vi "Limits Page.vi"(8 "error in (no error)":errorcluster, 10 "LBCB Number":T2) -> (0 "error out":errorcluster)   [LabVIEW 2009]
uses:
  lib/Limits/Limit Slider.ctl
  lib/Data Access Objects/Metadata/LBCB Number.ctl
  lib/Data Access Objects/Limits/DofTypes.ctl
  lib/Limits/Slider Messages.ctl
  lib/Control Loop/Parameters Changes.ctl
  lib/Control Loop/Parameter Change States.ctl
  lib/Data Access Objects/Metadata/Persistant DAO Actions.ctl
  lib/Data Access Objects/Application/Number Of LBCBs.ctl
  lib/Limits/Faults List Actions.ctl
  lib/Limits/Lower Upper Select.ctl
  lib/Launcher/NoPanelAppTypes.ctl
  lib/Launcher/Launcher Actions.ctl
panel:
  out "Messages":string
  in  "Ok":bool
  in  "DofType":T1
  in  "Limit Slider 6":T3 {"Slide" scale=-0.3..0.3 scale format="%#_6f"}
  in  "Limit Slider 5":T3 {"Slide" scale=-0.3..0.3 scale format="%#_6f"}
  in  "Limit Slider 4":T3 {"Slide" scale=-0.3..0.3 scale format="%#_6f"}
  in  "Limit Slider 3":T3 {"Slide" scale=-1.0..1.0 scale format="%#_6f"}
  in  "Limit Slider 2":T3 {"Slide" scale=-1.0..1.0 scale format="%#_6f"}
  in  "Limit Slider 1":T3 {"Slide" scale=-1.0..1.0 scale format="%#_6f"}
  # "Lower"
  # "Higher"
  # "Current"
  # "Global"
  # "Local"
  # "Lower"
  # "Higher"
  # "Current"
  # "Global"
  # "Local"
  # "Lower"
  # "Higher"
  # "Current"
  # "Global"
  # "Local"
  # "Lower"
  # "Higher"
  # "Current"
  # "Global"
  # "Local"
  # "Lower"
  # "Higher"
  # "Current"
  # "Global"
  # "Local"
  # "Lower"
  # "Higher"
  # "Current"
  # "Global"
  # "Local"
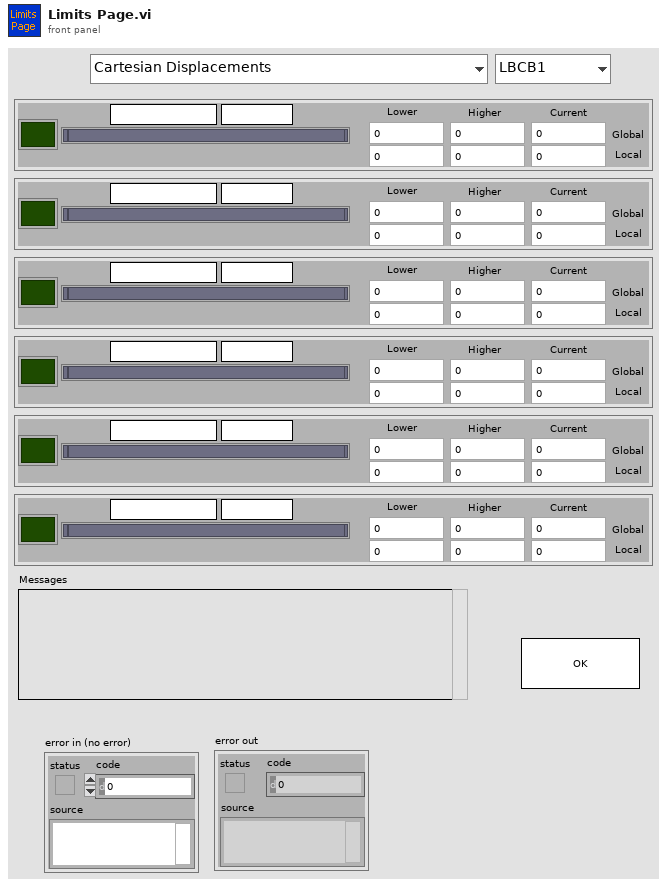
[diagram p1: front panel]
types:
  T1 = typedef "DofTypes.ctl" = enum16{"Cartesian Displacements", "Cartesian Forces & Moments", "Actuator Displacements", "Actuator Forces"}
  T2 = typedef "LBCB Number.ctl" = enum16{"LBCB1", "LBCB2"}
  T3 = typedef "Limit Slider.ctl" = cluster{"Slide":cluster{dbl, dbl, dbl, dbl}, "Global Lo":dbl, "Global Hi":dbl, "Local Lo":dbl, "Local Hi":dbl, "Fault":bool, "DofLabel":string, "Units":string, "Global Actual":dbl, "Local Actual":dbl}
  T4 = typedef "Parameters Changes.ctl" = cluster{"Change State":T5, "LBCB Number":T2}
  T5 = typedef "Parameter Change States.ctl" = enum16{"Mixed Mode", "Control Loop", "Limits", "Application", "Stiffness Jacobian", "Start DAQ", "Reset Auto-Balance", "Set Command", "Enable Control", "Disable Control", "Position", "Stop Application"}
  T6 = typedef "Slider Messages.ctl" = enum16{"Update Display", "Exit", "Nothing"}
  T7 = typedef "Persistant DAO Actions.ctl" = enum16{"Init", "Get", "Set", "Load", "Save"}
  T8 = enum8{"Enabled", "Disabled", "Disabled and Grayed Out"}
  T9 = typedef "Number Of LBCBs.ctl" = enum16{"1", "2"}
  T10 = typedef "Faults List Actions.ctl" = enum16{"Init", "Add", "Remove", "Get List"}
  T11 = typedef "Lower Upper Select.ctl" = enum16{"Lower", "Upper"}
  T12 = typedef "Fault Id.ctl" = cluster{"Fault Type":T13, "LBCB Number":T2, "Index":u32, "Space Type":T14}
  T13 = typedef "Fault Type.ctl" = enum16{"None", "Command", "Displacement", "Force", "Increment"}
  T14 = typedef "Space Type.ctl" = enum16{"Actuator", "Cartesian"}
  T15 = cluster{"[0]":dbl, "[1]":dbl, "[2]":dbl, "[3]":dbl, "[4]":dbl, "[5]":dbl, "[6]":dbl, "[7]":dbl, "[8]":dbl}[]
  T16 = cluster{"[0]":dbl, "[1]":dbl, "[2]":dbl, "[3]":dbl, "[4]":dbl, "[5]":dbl, "[6]":dbl, "[7]":dbl, "[8]":dbl}
  T17 = cluster{"[0]":dbl, "[1]":dbl, "[2]":dbl, "[3]":dbl}
  T18 = typedef "NoPanelAppTypes.ctl" = enum16{"NTCP Socket", "Data Archiving", "DAQ Link", "Control Loops", "Cmd Disp Diffs", "Connection Offsets", "Limits", "Increment Limits"}
  T19 = typedef "Launcher Actions.ctl" = enum16{"Launch", "Stop All", "Stop", "Kill", "Running?", "Init"}
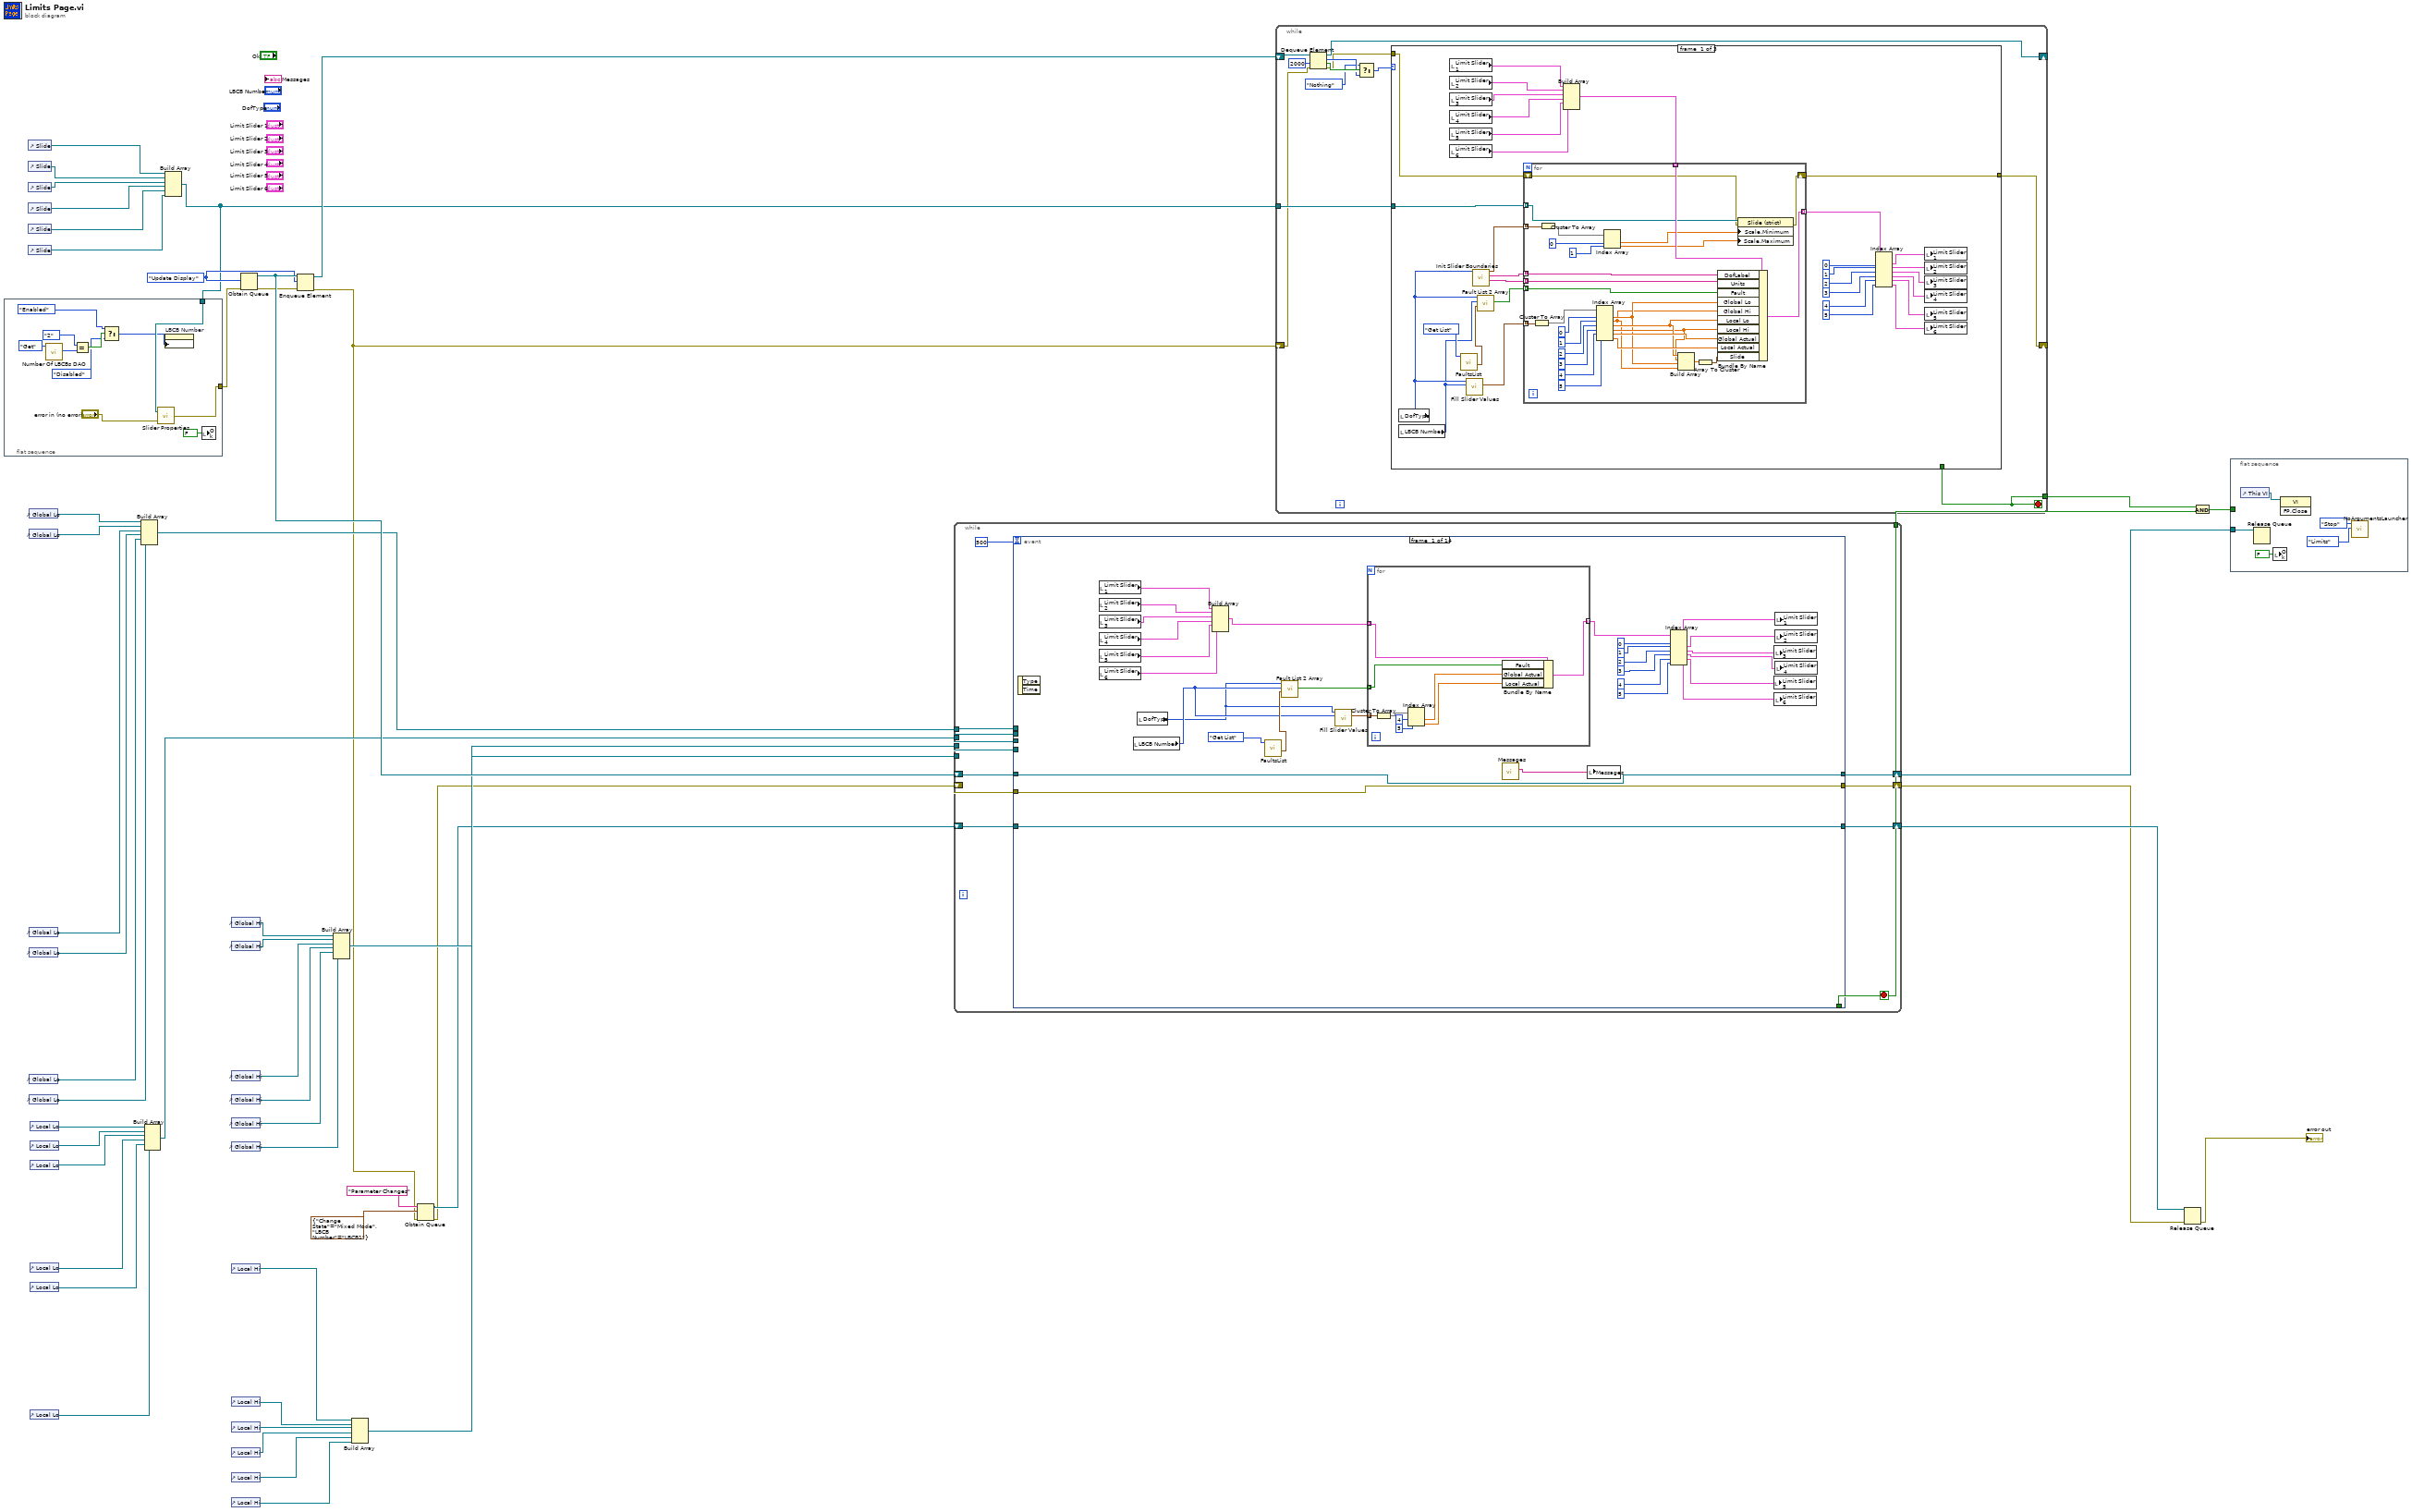
[diagram p0: block diagram]
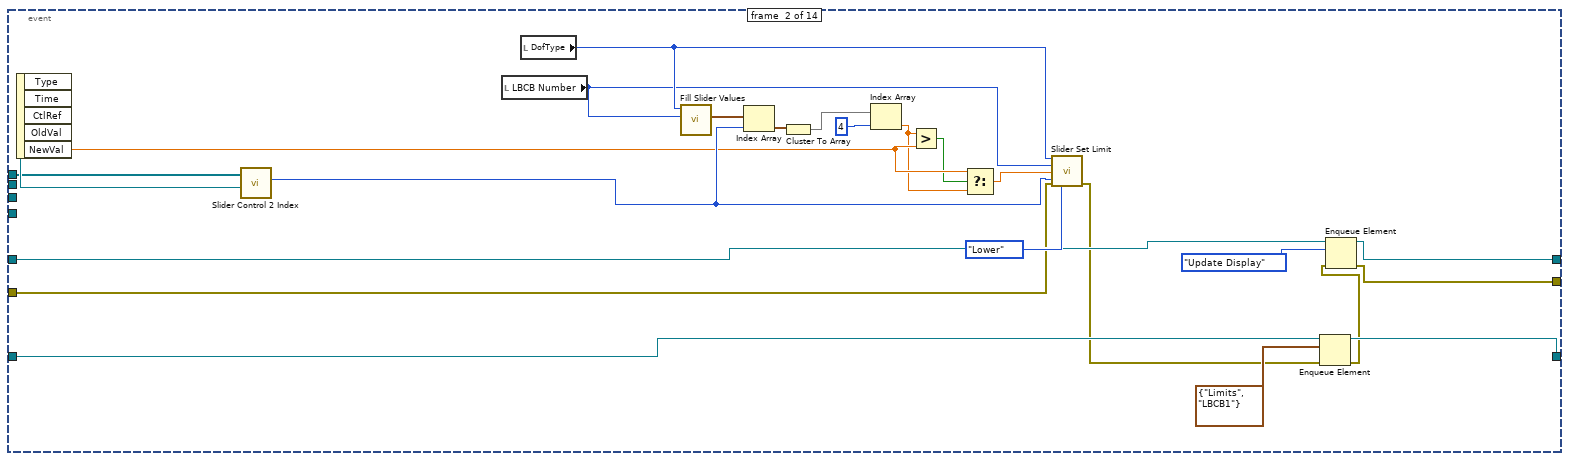
[diagram p2: hidden frame]
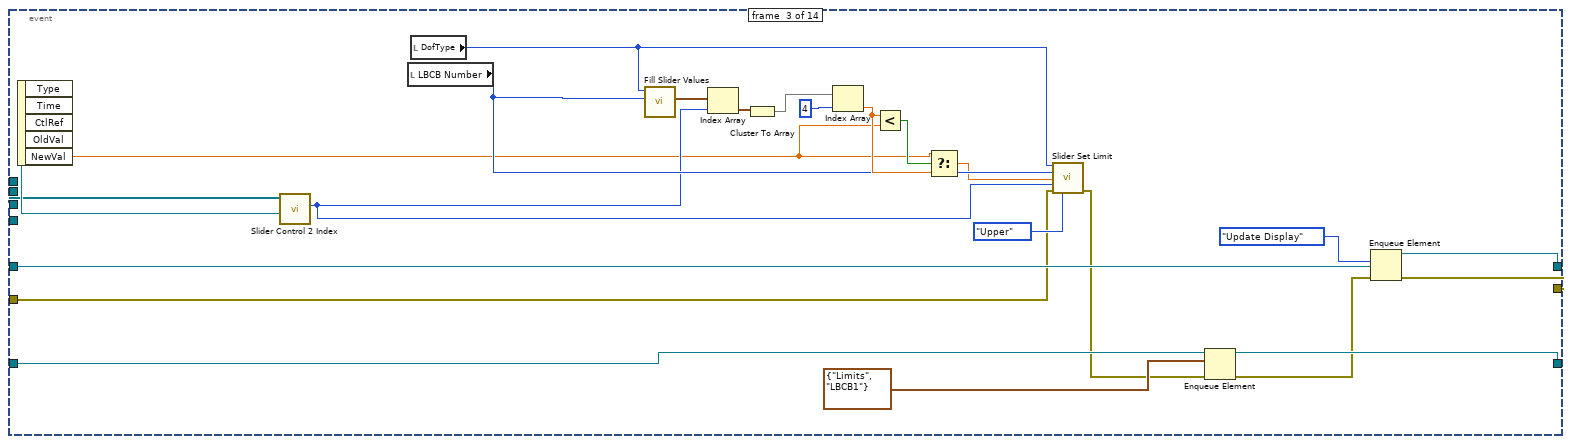
[diagram p3: hidden frame]
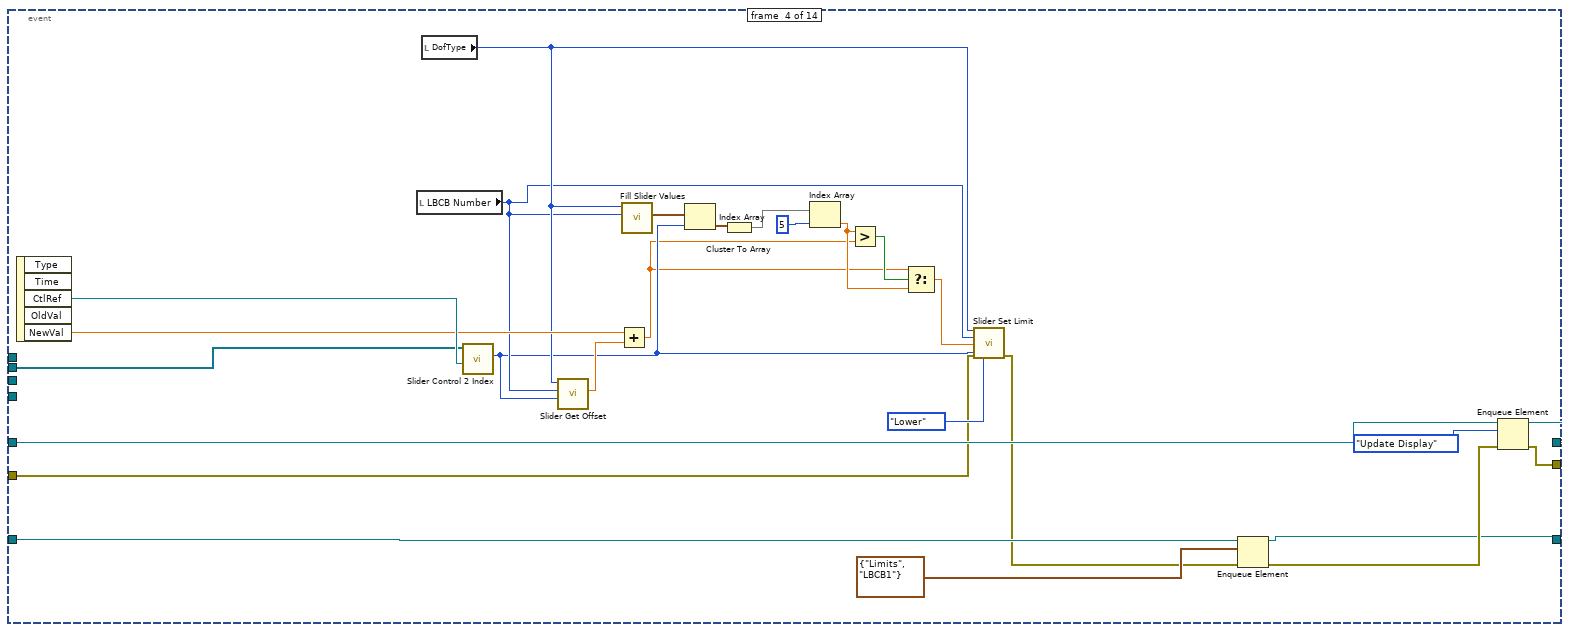
[diagram p4: hidden frame]
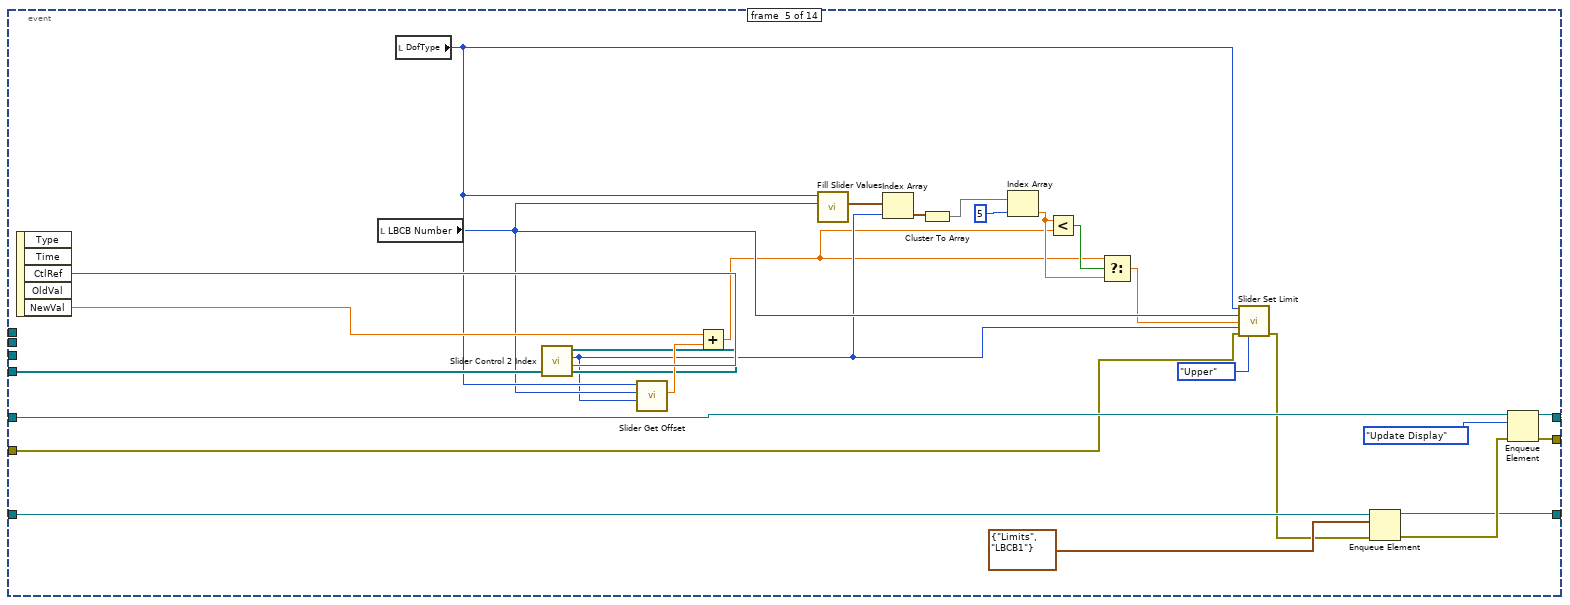
[diagram p5: hidden frame]
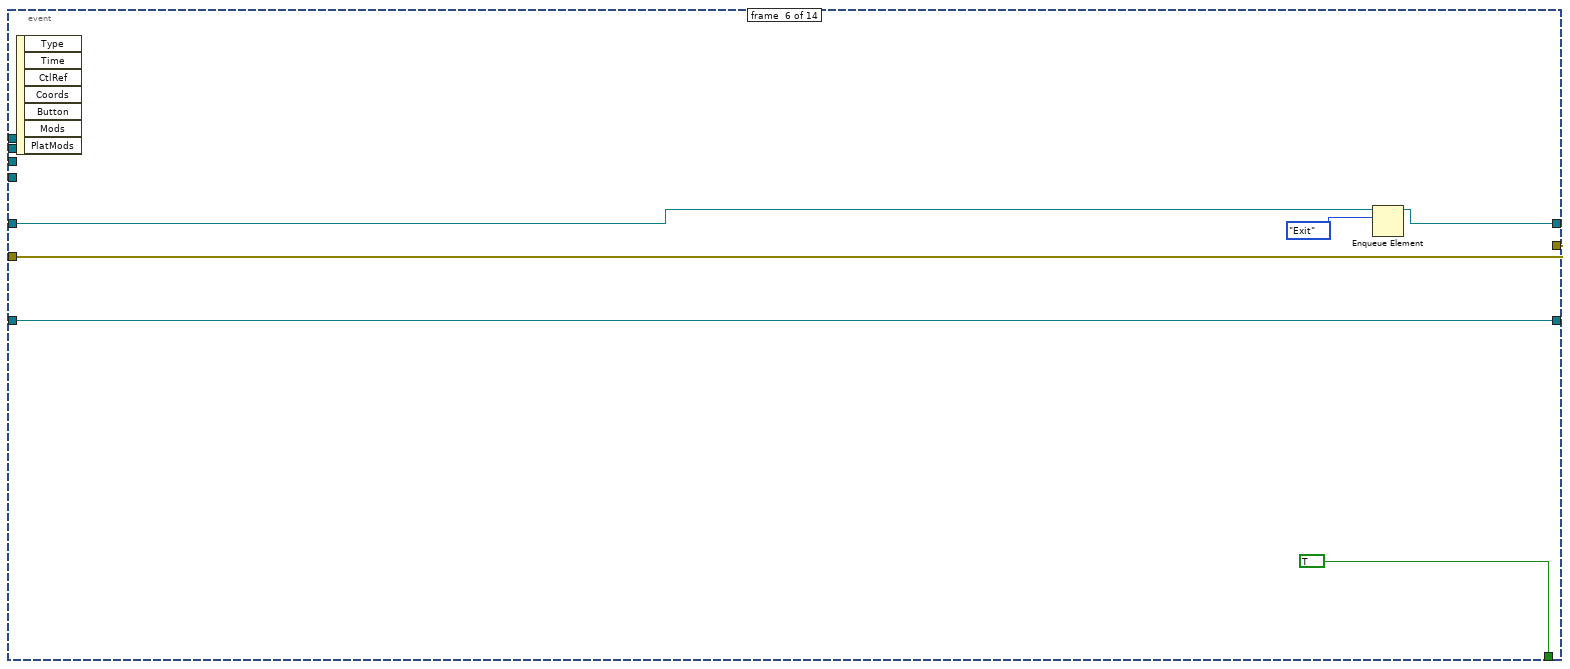
[diagram p6: hidden frame]
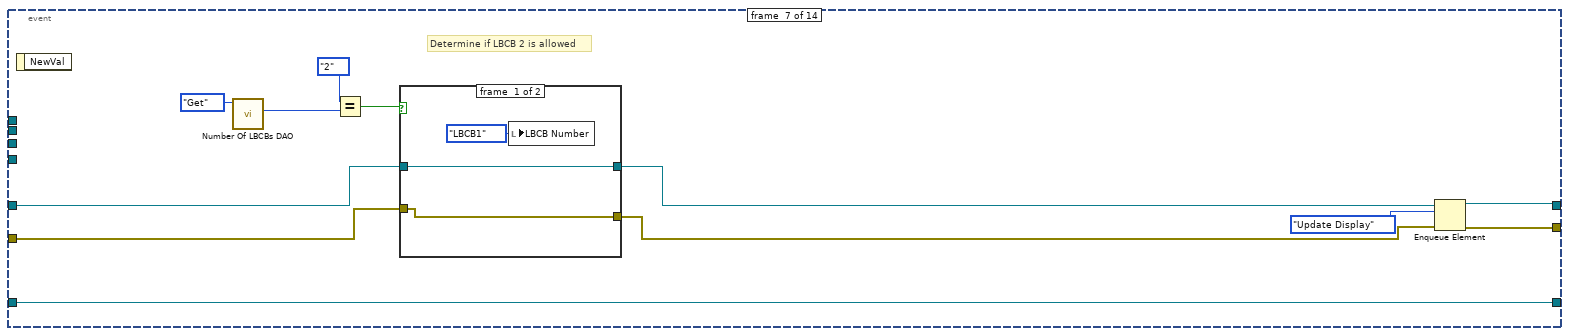
[diagram p7: hidden frame]
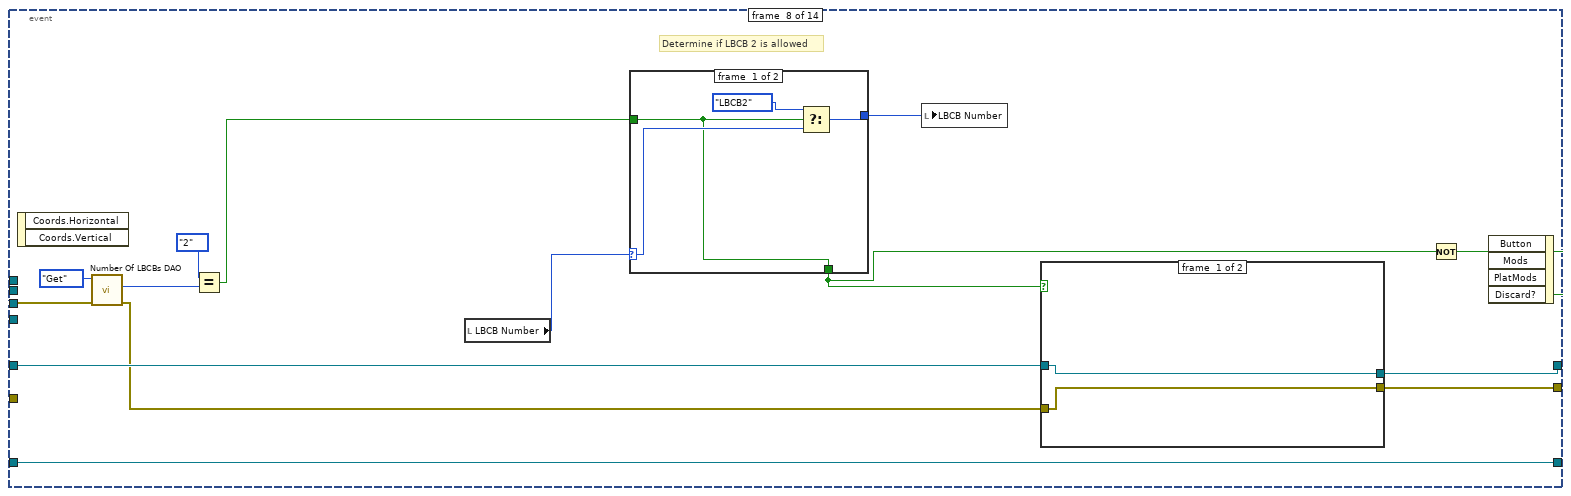
[diagram p9: hidden frame]
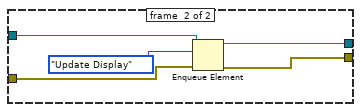
[diagram p10: hidden frame]
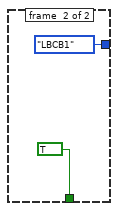
[diagram p11: hidden frame]
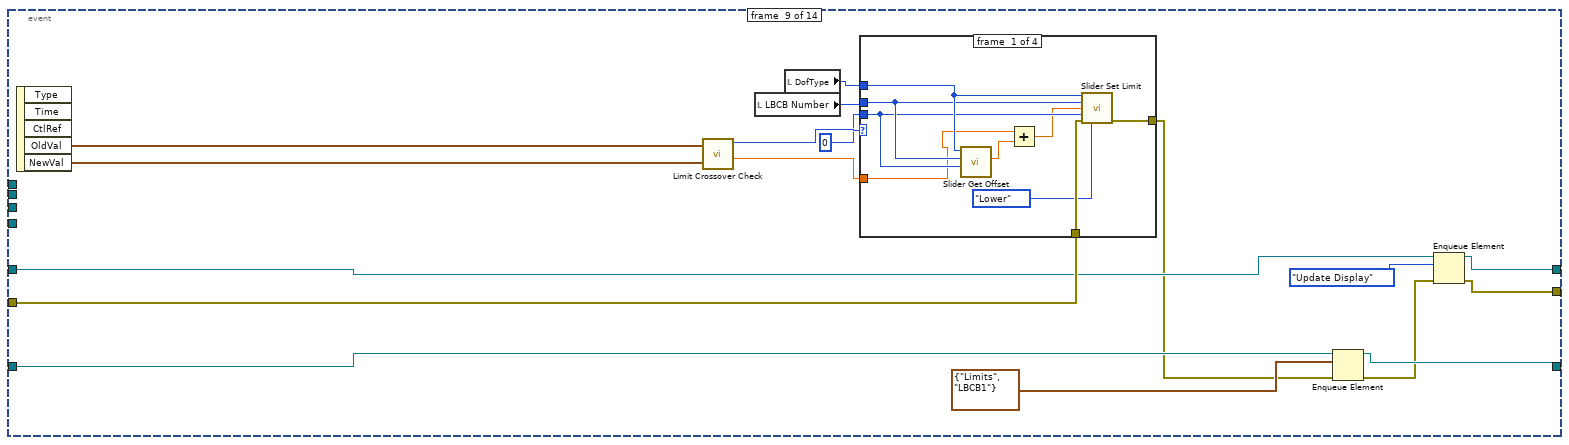
[diagram p12: hidden frame]
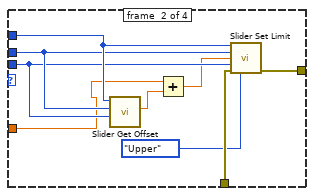
[diagram p13: hidden frame]
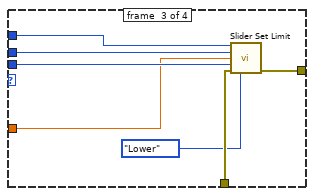
[diagram p14: hidden frame]
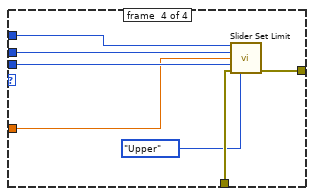
[diagram p15: hidden frame]
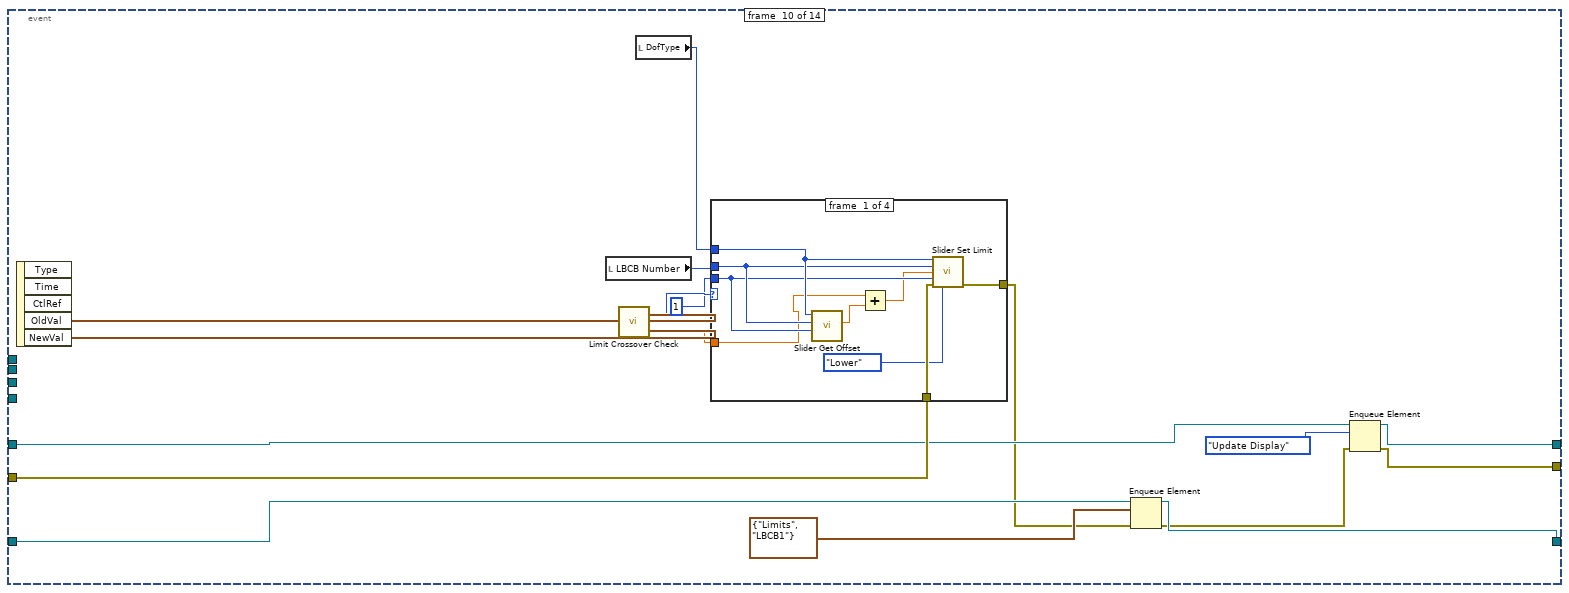
[diagram p16: hidden frame]
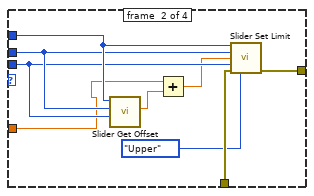
[diagram p17: hidden frame]
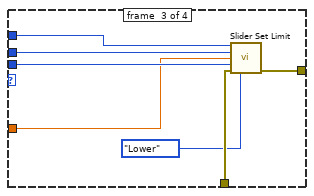
[diagram p18: hidden frame]
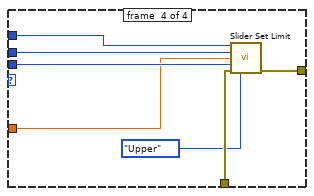
[diagram p19: hidden frame]
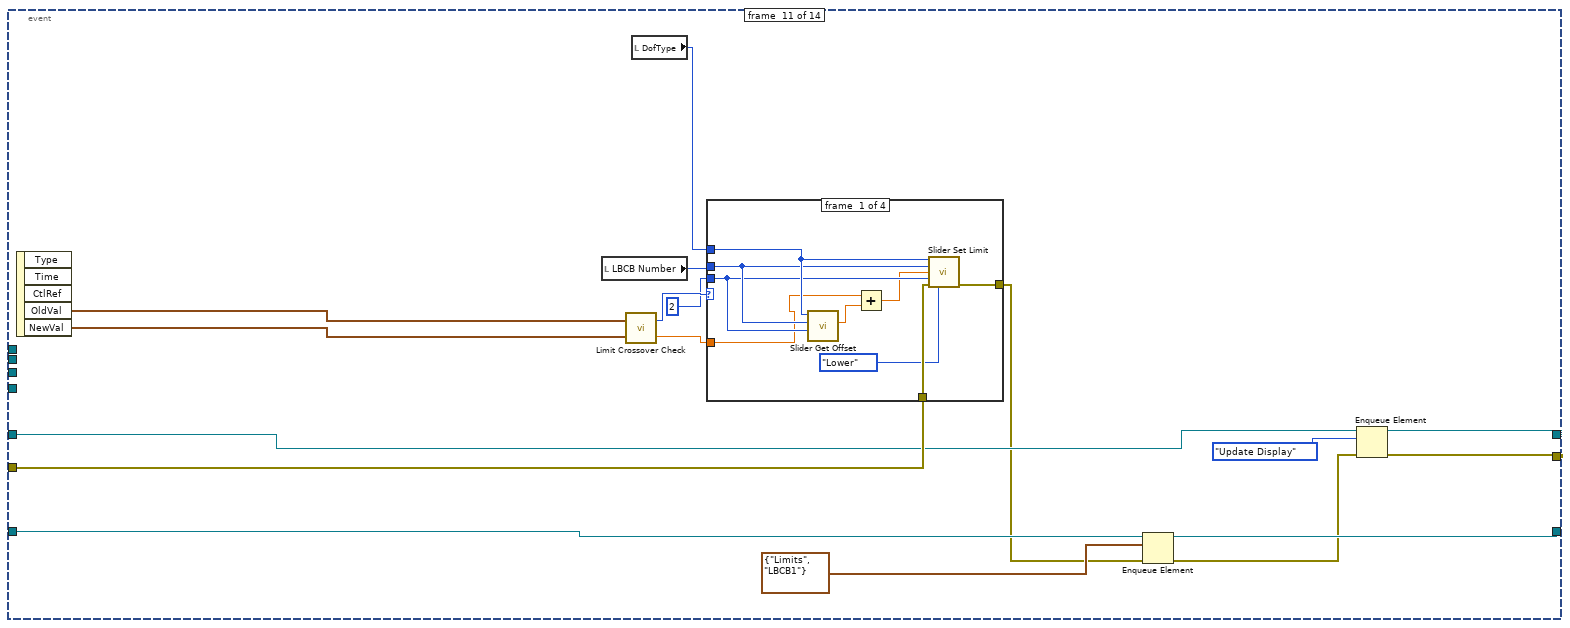
[diagram p20: hidden frame]
diagram:
  w47 = Slider_Messages."Update Display" ("Slider Message")
  n1 = flat-sequence {
    tunnel: w12 -> [w62]
    tunnel: [w61] -> w11
    frame #0 {
      n2 = call "Number Of LBCBs DAO.vi"("Actions"=Persistant_DAO_Actions."Get") -> ("Number of\nLBCBs Out"=w60:T9)  [unwired: 7 in, 3 out]
      n3 = Equal?(x=Number_Of_LBCBs."2", y=w60) -> (x = y?=w58:bool)
      n4 = Select(t=T8."Enabled" ("Disabled"), s=w58, f=T8."Disabled") -> (s? t:f=w55:T8)
      n5 = call "Slider Properties.vi"("error in (no error) 2"="error in (no error)", "Array"=w62) -> ("error out"=w61:errorcluster)
      n6 = property on="LBCB Number" class="Enum (strict)"("DisabledEnum"=w55) -> ()  [unwired: 2 in, 2 out]
      n7 = local write "Ok"(FALSE ("Ok")) -> ()
    }
  }
  n8 = control-ref of="Slide"() -> (w46:refnum<vi>)
  n9 = control-ref of="Slide"() -> (w45:refnum<vi>)
  n10 = control-ref of="Slide"() -> (w44:refnum<vi>)
  n11 = control-ref of="Slide"() -> (w43:refnum<vi>)
  n12 = control-ref of="Slide"() -> (w42:refnum<vi>)
  n13 = control-ref of="Slide"() -> (w41:refnum<vi>)
  n14 = control-ref of="Global Lo"() -> (w40:refnum<vi>)
  n15 = control-ref of="Global Lo"() -> (w39:refnum<vi>)
  n16 = control-ref of="Global Lo"() -> (w38:refnum<vi>)
  n17 = control-ref of="Global Lo"() -> (w37:refnum<vi>)
  n18 = control-ref of="Global Lo"() -> (w36:refnum<vi>)
  n19 = control-ref of="Global Lo"() -> (w35:refnum<vi>)
  n20 = control-ref of="Local Lo"() -> (w34:refnum<vi>)
  n21 = control-ref of="Local Lo"() -> (w33:refnum<vi>)
  n22 = control-ref of="Local Lo"() -> (w32:refnum<vi>)
  n23 = control-ref of="Local Lo"() -> (w31:refnum<vi>)
  n24 = control-ref of="Local Lo"() -> (w30:refnum<vi>)
  n25 = control-ref of="Local Lo"() -> (w29:refnum<vi>)
  n26 = Build Array(w40, w39, w38, w37, w36, w35) -> (w14:refnum<vi>[])
  n27 = Build Array(w34, w33, w32, w31, w30, w29) -> (w15:refnum<vi>[])
  n28 = Build Array(w46, w45, w44, w43, w42, w41) -> (w12:refnum<vi>[])
  n29 = control-ref of="Global Hi"() -> (w28:refnum<vi>)
  n30 = control-ref of="Global Hi"() -> (w27:refnum<vi>)
  n31 = control-ref of="Global Hi"() -> (w26:refnum<vi>)
  n32 = control-ref of="Global Hi"() -> (w25:refnum<vi>)
  n33 = control-ref of="Global Hi"() -> (w24:refnum<vi>)
  n34 = control-ref of="Global Hi"() -> (w23:refnum<vi>)
  n35 = control-ref of="Local Hi"() -> (w22:refnum<vi>)
  n36 = control-ref of="Local Hi"() -> (w21:refnum<vi>)
  n37 = control-ref of="Local Hi"() -> (w9:refnum<vi>)
  n38 = control-ref of="Local Hi"() -> (w20:refnum<vi>)
  n39 = control-ref of="Local Hi"() -> (w19:refnum<vi>)
  n40 = control-ref of="Local Hi"() -> (w18:refnum<vi>)
  n41 = Obtain Queue(element data type=w47, error in (no error)=w11) -> (queue out=w52:refnum<queue>, error out=w13:errorcluster)  [unwired: 3 in, 1 out]
  n42 = Enqueue Element(queue=w52, element=w47, error in (no error)=w13) -> (queue out=w48:refnum<queue>, error out=w5:errorcluster)  [unwired: 1 in, 1 out]
  n43 = Build Array(w28, w27, w26, w25, w24, w23) -> (w16:refnum<vi>[])
  n44 = Build Array(w22, w21, w9, w20, w19, w18) -> (w17:refnum<vi>[])
  n45 = Obtain Queue(name (unnamed)="Parameter Changes", element data type=T4 {"Change State"=enum."Mixed Mode", "LBCB Number"=enum."LBCB1"} ("Parameter Changes"), error in (no error)=w5) -> (queue out=w6:refnum<queue>, error out=w4:errorcluster)  [unwired: 2 in, 1 out]
  n46 = while {
    shift-right: [w73] -> w10
    shift-left: w52 -> [w74]
    tunnel: [w72] -> w50
    tunnel: w17 -> [w69]
    tunnel: w16 -> [w68]
    tunnel: w15 -> [w70]
    tunnel: w14 -> [w71]
    shift-right: [w66] -> w2
    shift-left: w4 -> [w67]
    shift-right: [w64] -> w3
    shift-left: w6 -> [w65]
    stop <- w72 stop-if-true
    n47 = event shown="[5] \"Ok\": Mouse Down" {
      selector: _ -> [_ _ _ _ _ _ _ _ _ _ _ _ _ _]
      dyn-events: _ -> [_ _ _ _ _ _ _ _ _ _ _ _ _ _]
      timeout: 500 -> [_ _ _ _ _ _ _ _ _ _ _ _ _ _]
      tunnel: w74 -> [w104 w135 w159 w183 w210 w219 w225 w251 w272 w321 w370 w421 w468 w517]
      tunnel: [w104 w134 w158 w182 w208 w218 w231 w250 w271 w320 w369 w420 w467 w516] -> w73
      tunnel: [_ _ _ _ _ TRUE _ _ _ _ _ _ _ _] -> w72
      tunnel: w71 -> [_ w133 _ _ _ _ _ _ _ _ _ _ _ _]
      tunnel: w70 -> [_ _ _ w181 _ _ _ _ _ _ _ _ _ _]
      tunnel: w69 -> [_ _ _ _ w207 _ _ _ _ _ _ _ _ _]
      tunnel: w68 -> [_ _ w157 _ _ _ _ _ _ _ _ _ _ _]
      tunnel: w67 -> [w103 w132 w156 w180 w206 w216 w223 w247 w274 w323 w372 w423 w470 w519]
      tunnel: [w103 w131 w155 w179 w205 w216 w230 w249 w270 w319 w368 w419 w466 w515] -> w66
      tunnel: w65 -> [w102 w129 w153 w177 w203 w215 w229 w248 w268 w317 w366 w415 w464 w513]
      tunnel: [w102 w128 w152 w174 w200 w215 w229 w248 w267 w316 w364 w414 w463 w512] -> w64
      event #0 {
        n48 = event-data() -> ()  [unwired: 1 in, 2 out]
        n49 = local read "Limit Slider 1"() -> (w99:T3)
        n50 = local read "Limit Slider 2"() -> (w98:T3)
        n51 = local read "Limit Slider 3"() -> (w97:T3)
        n52 = local read "Limit Slider 4"() -> (w96:T3)
        n53 = local read "Limit Slider 5"() -> (w95:T3)
        n54 = local read "Limit Slider 6"() -> (w94:T3)
        n55 = local read "LBCB Number"() -> (w78:T2)
        n56 = local read "DofType"() -> (w77:T1)
        n57 = Build Array(w99, w98, w97, w96, w95, w94) -> (w86:T3[])
        n58 = call "FaultsList.vi"("Limits List Actions"=Faults_List_Actions."Get List") -> ("Fault List"=w100:T12[])  [unwired: 2 in, 8 out]
        n59 = call "Fault List 2 Array.vi"("Fault List"=w100, "LBCB Number"=w78, "DofType"=w77) -> ("Faults"=w87:bool[])  [unwired: 8 in]
        n60 = call "Fill Slider Values.vi"("LBCB Number"=w78, "DofType"=w77) -> ("Silder Values"=w76:T15)  [unwired: 9 in]
        n61 = for {
          tunnel: w87 -> [w113] mode=indexing
          tunnel: w86 -> [w114] mode=indexing
          tunnel: [w112] -> w85 mode=indexing
          tunnel: w76 -> [w111] mode=indexing
          n62 = Cluster To Array(cluster=w111) -> (array=w110:dbl[])
          n63 = Index Array(array=w110, index #1=4 ("index"), index #2=5 ("index")) -> (element #1=w107:dbl, element #2=w106:dbl)
          n64 = Bundle By Name(cluster=w114, "Fault"=w113, "Global Actual"=w107, "Local Actual"=w106) -> (w112:T3)
        }
        n65 = call "Messages.vi"() -> ("Messages"=w105:string)  [unwired: 2 in, 9 out]
        n66 = local write "Messages"(w105) -> ()
        n67 = Index Array(array=w85, index #1=0 ("index"), index #2=1 ("index"), index #3=2 ("index"), index #4=3 ("index"), index #5=4 ("index"), index #6=5 ("index")) -> (element #1=w84:T3, element #2=w83:T3, element #3=w82:T3, element #4=w81:T3, element #5=w80:T3, element #6=w79:T3)
        n68 = local write "Limit Slider 5"(w80) -> ()
        n69 = local write "Limit Slider 3"(w82) -> ()
        n70 = local write "Limit Slider 6"(w79) -> ()
        n71 = local write "Limit Slider 1"(w84) -> ()
        n72 = local write "Limit Slider 2"(w83) -> ()
        n73 = local write "Limit Slider 4"(w81) -> ()
      }
      event #1 {
        n74 = event-data() -> ("CtlRef"=w138:refnum<vi>, "NewVal"=w118:dbl)  [unwired: 1 in, 3 out]
        n75 = call "Slider Control 2 Index.vi"("Control"=w138, "Controls"=w133) -> ("Index"=w122:i32)  [unwired: 9 in]
        n76 = local read "LBCB Number"() -> (w124:T2)
        n77 = local read "DofType"() -> (w125:T1)
        n78 = call "Fill Slider Values.vi"("LBCB Number"=w124, "DofType"=w125) -> ("Silder Values"=w123:T15)  [unwired: 9 in]
        n79 = Index Array(array=w123, index=w122) -> (element=w121:T16)
        n80 = Cluster To Array(cluster=w121) -> (array=w120:dbl[])
        n81 = Index Array(array=w120, index=4) -> (element=w115:dbl)
        n82 = Greater?(x=w115, y=w118) -> (0:w116:bool)
        n83 = Select(t=w118, s=w116, f=w115) -> (s? t:f=w117:dbl)
        n84 = call "Slider Set Limit.vi"("DofType"=w125, "LBCB Number"=w124, "Value"=w117, "Index"=w122, "error in (no error)"=w132, "Lower/Upper"=Lower_Upper_Select."Lower") -> ("error out"=w127:errorcluster)  [unwired: 9 in]
        n85 = Enqueue Element(queue=w129, element=T4 {"Change State"=enum."Limits", "LBCB Number"=enum."LBCB1"}, error in (no error)=w127) -> (queue out=w128:refnum<queue>, error out=w126:errorcluster)  [unwired: 2 out]
        n86 = Enqueue Element(queue=w135, element=Slider_Messages."Update Display", error in (no error)=w126) -> (queue out=w134:refnum<queue>, error out=w131:errorcluster)  [unwired: 1 in, 1 out]
      }
      event #2 {
        n87 = event-data() -> ("CtlRef"=w162:refnum<vi>, "NewVal"=w139:dbl)  [unwired: 1 in, 3 out]
        n88 = call "Slider Control 2 Index.vi"("Control"=w162, "Controls"=w157) -> ("Index"=w141:i32)  [unwired: 9 in]
        n89 = local read "LBCB Number"() -> (w142:T2)
        n90 = local read "DofType"() -> (w143:T1)
        n91 = call "Fill Slider Values.vi"("LBCB Number"=w142, "DofType"=w143) -> ("Silder Values"=w149:T15)  [unwired: 9 in]
        n92 = Index Array(array=w149, index=w141) -> (element=w148:T16)
        n93 = Cluster To Array(cluster=w148) -> (array=w147:dbl[])
        n94 = Index Array(array=w147, index=4) -> (element=w144:dbl)
        n95 = Less?(x=w144, y=w139) -> (x < y?=w145:bool)
        n96 = Select(t=w139, s=w145, f=w144) -> (s? t:f=w140:dbl)
        n97 = call "Slider Set Limit.vi"("DofType"=w143, "LBCB Number"=w142, "Value"=w140, "Index"=w141, "error in (no error)"=w156, "Lower/Upper"=Lower_Upper_Select."Upper") -> ("error out"=w151:errorcluster)  [unwired: 9 in]
        n98 = Enqueue Element(queue=w153, element=T4 {"Change State"=enum."Limits", "LBCB Number"=enum."LBCB1"}, error in (no error)=w151) -> (queue out=w152:refnum<queue>, error out=w150:errorcluster)  [unwired: 2 out]
        n99 = Enqueue Element(queue=w159, element=Slider_Messages."Update Display", error in (no error)=w150) -> (queue out=w158:refnum<queue>, error out=w155:errorcluster)  [unwired: 1 in, 1 out]
      }
      event #3 {
        n100 = event-data() -> ("CtlRef"=w188:refnum<vi>, "NewVal"=w186:dbl)  [unwired: 1 in, 3 out]
        n101 = local read "LBCB Number"() -> (w166:T2)
        n102 = local read "DofType"() -> (w167:T1)
        n103 = call "Slider Control 2 Index.vi"("Control"=w188, "Controls"=w181) -> ("Index"=w165:i32)  [unwired: 9 in]
        n104 = call "Slider Get Offset.vi"("Index"=w165, "LBCB Number"=w166, "DofType"=w167) -> ("Offset"=w185:dbl)  [unwired: 8 in]
        n105 = Add(x=w186, y=w185) -> (x+y=w164:dbl)
        n106 = call "Fill Slider Values.vi"("LBCB Number"=w166, "DofType"=w167) -> ("Silder Values"=w173:T15)  [unwired: 9 in]
        n107 = Index Array(array=w173, index=w165) -> (element=w172:T16)
        n108 = Cluster To Array(cluster=w172) -> (array=w171:dbl[])
        n109 = Index Array(array=w171, index=5) -> (element=w168:dbl)
        n110 = Greater?(x=w168, y=w164) -> (0:w169:bool)
        n111 = Select(t=w164, s=w169, f=w168) -> (s? t:f=w163:dbl)
        n112 = call "Slider Set Limit.vi"("DofType"=w167, "LBCB Number"=w166, "Value"=w163, "Index"=w165, "error in (no error)"=w180, "Lower/Upper"=Lower_Upper_Select."Lower") -> ("error out"=w176:errorcluster)  [unwired: 9 in]
        n113 = Enqueue Element(queue=w177, element=T4 {"Change State"=enum."Limits", "LBCB Number"=enum."LBCB1"}, error in (no error)=w176) -> (queue out=w174:refnum<queue>, error out=w175:errorcluster)  [unwired: 2 out]
        n114 = Enqueue Element(queue=w183, element=Slider_Messages."Update Display", error in (no error)=w175) -> (queue out=w182:refnum<queue>, error out=w179:errorcluster)  [unwired: 1 in, 1 out]
      }
      event #4 {
        n115 = event-data() -> ("CtlRef"=w214:refnum<vi>, "NewVal"=w212:dbl)  [unwired: 1 in, 3 out]
        n116 = local read "LBCB Number"() -> (w192:T2)
        n117 = local read "DofType"() -> (w193:T1)
        n118 = call "Slider Control 2 Index.vi"("Control"=w214, "Controls"=w207) -> ("Index"=w191:i32)  [unwired: 9 in]
        n119 = call "Slider Get Offset.vi"("Index"=w191, "LBCB Number"=w192, "DofType"=w193) -> ("Offset"=w211:dbl)  [unwired: 8 in]
        n120 = Add(x=w212, y=w211) -> (x+y=w190:dbl)
        n121 = call "Fill Slider Values.vi"("LBCB Number"=w192, "DofType"=w193) -> ("Silder Values"=w199:T15)  [unwired: 9 in]
        n122 = Index Array(array=w199, index=w191) -> (element=w198:T16)
        n123 = Cluster To Array(cluster=w198) -> (array=w197:dbl[])
        n124 = Index Array(array=w197, index=5) -> (element=w194:dbl)
        n125 = Less?(x=w194, y=w190) -> (x < y?=w195:bool)
        n126 = Select(t=w190, s=w195, f=w194) -> (s? t:f=w189:dbl)
        n127 = call "Slider Set Limit.vi"("DofType"=w193, "LBCB Number"=w192, "Value"=w189, "Index"=w191, "error in (no error)"=w206, "Lower/Upper"=Lower_Upper_Select."Upper") -> ("error out"=w202:errorcluster)  [unwired: 9 in]
        n128 = Enqueue Element(queue=w203, element=T4 {"Change State"=enum."Limits", "LBCB Number"=enum."LBCB1"}, error in (no error)=w202) -> (queue out=w200:refnum<queue>, error out=w201:errorcluster)  [unwired: 2 out]
        n129 = Enqueue Element(queue=w210, element=Slider_Messages."Update Display", error in (no error)=w201) -> (queue out=w208:refnum<queue>, error out=w205:errorcluster)  [unwired: 1 in, 1 out]
      }
      event #5 {
        n130 = event-data() -> ()  [unwired: 1 in, 7 out]
        n131 = Enqueue Element(queue=w219, element=Slider_Messages."Exit") -> (queue out=w218:refnum<queue>)  [unwired: 2 in, 2 out]
      }
      event #6 {
        # "Determine if LBCB 2 is allowed"
        n132 = event-data() -> ()  [unwired: 1 in, 1 out]
        n133 = call "Number Of LBCBs DAO.vi"("Actions"=Persistant_DAO_Actions."Get") -> ("Number of\nLBCBs Out"=w227:T9)  [unwired: 7 in, 3 out]
        n134 = Equal?(x=Number_Of_LBCBs."2", y=w227) -> (x = y?=w221:bool)
        n135 = case shown="False" w221 {
          tunnel: w225 -> [w235 w237]
          tunnel: [w235 w237] -> w224
          tunnel: w223 -> [w234 w236]
          tunnel: [w234 w236] -> w222
          frame #0 {
            n136 = local write "LBCB Number"(LBCB_Number."LBCB1" ("LBCB Number")) -> ()
          }
          frame #1 {
          }
        }
        n137 = Enqueue Element(queue=w224, element=Slider_Messages."Update Display", error in (no error)=w222) -> (queue out=w231:refnum<queue>, error out=w230:errorcluster)  [unwired: 1 in, 1 out]
      }
      event #7 {
        # "Determine if LBCB 2 is allowed"
        n138 = event-data() -> ()  [unwired: 1 in, 2 out]
        n139 = call "Number Of LBCBs DAO.vi"("error in (no error)"=w247, "Actions"=Persistant_DAO_Actions."Get") -> ("error out"=w245:errorcluster, "Number of\nLBCBs Out"=w244:T9)  [unwired: 6 in, 2 out]
        n140 = Equal?(x=Number_Of_LBCBs."2", y=w244) -> (x = y?=w238:bool)
        n141 = local read "LBCB Number"() -> (w242:T2)
        n142 = case shown="\"LBCB1\", Default" w242 {
          selector: w242 -> [w261 _]
          tunnel: [w262 LBCB_Number."LBCB1" ("LBCB Number")] -> w241
          tunnel: w238 -> [w259 _]
          tunnel: [w259 TRUE] -> w240
          frame #0 {
            n143 = Select(t=LBCB_Number."LBCB2", s=w259, f=w261) -> (s? t:f=w262:T2)
          }
          frame #1 {
          }
        }
        n144 = local write "LBCB Number"(w241) -> ()
        n145 = case shown="False" w240 {
          tunnel: w251 -> [w253 w258]
          tunnel: [w253 w257] -> w250
          tunnel: [w252 w256] -> w249
          tunnel: w245 -> [w252 w255]
          frame #0 {
          }
          frame #1 {
            n146 = Enqueue Element(queue=w258, element=Slider_Messages."Update Display", error in (no error)=w255) -> (queue out=w257:refnum<queue>, error out=w256:errorcluster)  [unwired: 1 in, 1 out]
          }
        }
        n147 = Not(x=w240) -> (.not. x?=w239:bool)
        n148 = event-data("Discard?"=w239) -> ()  [unwired: 4 in, 1 out]
      }
      event #8 {
        n149 = event-data() -> ("OldVal"=w281:cluster{dbl, dbl, dbl, dbl}, "NewVal"=w280:cluster{dbl, dbl, dbl, dbl})  [unwired: 1 in, 3 out]
        n150 = call "Limit Crossover Check.vi"("NewVal"=w280, "OldVal"=w281) -> ("Value"=w276:dbl, "Index"=w277:i32)
        n151 = local read "LBCB Number"() -> (w278:T2)
        n152 = local read "DofType"() -> (w279:T1)
        n153 = case shown="0, Default" w277 {
          tunnel: w279 -> [w290 w299 w306 w313]
          tunnel: w278 -> [w289 w298 w305 w312]
          tunnel: w276 -> [w286 w295 w300 w307]
          tunnel: 0 ("Index") -> [w288 w297 w304 w311]
          tunnel: w274 -> [w284 w293 w303 w310]
          tunnel: [w283 w292 w302 w309] -> w266
          frame #0 {
            n154 = call "Slider Get Offset.vi"("Index"=w288, "LBCB Number"=w289, "DofType"=w290) -> ("Offset"=w285:dbl)  [unwired: 8 in]
            n155 = Add(x=w286, y=w285) -> (x+y=w287:dbl)
            n156 = call "Slider Set Limit.vi"("DofType"=w290, "LBCB Number"=w289, "Value"=w287, "Index"=w288, "error in (no error)"=w284, "Lower/Upper"=Lower_Upper_Select."Lower") -> ("error out"=w283:errorcluster)  [unwired: 9 in]
          }
          frame #1 {
            n157 = call "Slider Get Offset.vi"("Index"=w297, "LBCB Number"=w298, "DofType"=w299) -> ("Offset"=w294:dbl)  [unwired: 8 in]
            n158 = Add(x=w295, y=w294) -> (x+y=w296:dbl)
            n159 = call "Slider Set Limit.vi"("DofType"=w299, "LBCB Number"=w298, "Value"=w296, "Index"=w297, "error in (no error)"=w293, "Lower/Upper"=Lower_Upper_Select."Upper") -> ("error out"=w292:errorcluster)  [unwired: 9 in]
          }
          frame #2 {
            n160 = call "Slider Set Limit.vi"("DofType"=w306, "LBCB Number"=w305, "Value"=w300, "Index"=w304, "error in (no error)"=w303, "Lower/Upper"=Lower_Upper_Select."Lower") -> ("error out"=w302:errorcluster)  [unwired: 9 in]
          }
          frame #3 {
            n161 = call "Slider Set Limit.vi"("DofType"=w313, "LBCB Number"=w312, "Value"=w307, "Index"=w311, "error in (no error)"=w310, "Lower/Upper"=Lower_Upper_Select."Upper") -> ("error out"=w309:errorcluster)  [unwired: 9 in]
          }
        }
        n162 = Enqueue Element(queue=w268, element=T4 {"Change State"=enum."Limits", "LBCB Number"=enum."LBCB1"}, error in (no error)=w266) -> (queue out=w267:refnum<queue>, error out=w265:errorcluster)  [unwired: 2 out]
        n163 = Enqueue Element(queue=w272, element=Slider_Messages."Update Display", error in (no error)=w265) -> (queue out=w271:refnum<queue>, error out=w270:errorcluster)  [unwired: 1 in, 1 out]
      }
      event #9 {
        n164 = event-data() -> ("OldVal"=w330:cluster{dbl, dbl, dbl, dbl}, "NewVal"=w329:cluster{dbl, dbl, dbl, dbl})  [unwired: 1 in, 3 out]
        n165 = local read "LBCB Number"() -> (w327:T2)
        n166 = call "Limit Crossover Check.vi"("NewVal"=w329, "OldVal"=w330) -> ("Value"=w325:dbl, "Index"=w326:i32)
        n167 = local read "DofType"() -> (w328:T1)
        n168 = case shown="0, Default" w326 {
          tunnel: w328 -> [w339 w348 w355 w362]
          tunnel: w327 -> [w338 w347 w354 w361]
          tunnel: w325 -> [w335 w344 w349 w356]
          tunnel: 1 ("Index") -> [w337 w346 w353 w360]
          tunnel: w323 -> [w333 w342 w352 w359]
          tunnel: [w332 w341 w351 w358] -> w315
          frame #0 {
            n169 = call "Slider Get Offset.vi"("Index"=w337, "LBCB Number"=w338, "DofType"=w339) -> ("Offset"=w334:dbl)  [unwired: 8 in]
            n170 = Add(x=w335, y=w334) -> (x+y=w336:dbl)
            n171 = call "Slider Set Limit.vi"("DofType"=w339, "LBCB Number"=w338, "Value"=w336, "Index"=w337, "error in (no error)"=w333, "Lower/Upper"=Lower_Upper_Select."Lower") -> ("error out"=w332:errorcluster)  [unwired: 9 in]
          }
          frame #1 {
            n172 = call "Slider Get Offset.vi"("Index"=w346, "LBCB Number"=w347, "DofType"=w348) -> ("Offset"=w343:dbl)  [unwired: 8 in]
            n173 = Add(x=w344, y=w343) -> (x+y=w345:dbl)
            n174 = call "Slider Set Limit.vi"("DofType"=w348, "LBCB Number"=w347, "Value"=w345, "Index"=w346, "error in (no error)"=w342, "Lower/Upper"=Lower_Upper_Select."Upper") -> ("error out"=w341:errorcluster)  [unwired: 9 in]
          }
          frame #2 {
            n175 = call "Slider Set Limit.vi"("DofType"=w355, "LBCB Number"=w354, "Value"=w349, "Index"=w353, "error in (no error)"=w352, "Lower/Upper"=Lower_Upper_Select."Lower") -> ("error out"=w351:errorcluster)  [unwired: 9 in]
          }
          frame #3 {
            n176 = call "Slider Set Limit.vi"("DofType"=w362, "LBCB Number"=w361, "Value"=w356, "Index"=w360, "error in (no error)"=w359, "Lower/Upper"=Lower_Upper_Select."Upper") -> ("error out"=w358:errorcluster)  [unwired: 9 in]
          }
        }
        n177 = Enqueue Element(queue=w317, element=T4 {"Change State"=enum."Limits", "LBCB Number"=enum."LBCB1"}, error in (no error)=w315) -> (queue out=w316:refnum<queue>, error out=w314:errorcluster)  [unwired: 2 out]
        n178 = Enqueue Element(queue=w321, element=Slider_Messages."Update Display", error in (no error)=w314) -> (queue out=w320:refnum<queue>, error out=w319:errorcluster)  [unwired: 1 in, 1 out]
      }
      event #10 {
        n179 = event-data() -> ("OldVal"=w379:cluster{dbl, dbl, dbl, dbl}, "NewVal"=w378:cluster{dbl, dbl, dbl, dbl})  [unwired: 1 in, 3 out]
        n180 = local read "LBCB Number"() -> (w376:T2)
        n181 = call "Limit Crossover Check.vi"("NewVal"=w378, "OldVal"=w379) -> ("Value"=w374:dbl, "Index"=w375:i32)
        n182 = local read "DofType"() -> (w377:T1)
        n183 = case shown="0, Default" w375 {
          tunnel: w377 -> [w388 w397 w404 w411]
          tunnel: w376 -> [w387 w396 w403 w410]
          tunnel: w374 -> [w384 w393 w398 w405]
          tunnel: 2 ("Index") -> [w386 w395 w402 w409]
          tunnel: w372 -> [w382 w391 w401 w408]
          tunnel: [w381 w390 w400 w407] -> w365
          frame #0 {
            n184 = call "Slider Get Offset.vi"("Index"=w386, "LBCB Number"=w387, "DofType"=w388) -> ("Offset"=w383:dbl)  [unwired: 8 in]
            n185 = Add(x=w384, y=w383) -> (x+y=w385:dbl)
            n186 = call "Slider Set Limit.vi"("DofType"=w388, "LBCB Number"=w387, "Value"=w385, "Index"=w386, "error in (no error)"=w382, "Lower/Upper"=Lower_Upper_Select."Lower") -> ("error out"=w381:errorcluster)  [unwired: 9 in]
          }
          frame #1 {
            n187 = call "Slider Get Offset.vi"("Index"=w395, "LBCB Number"=w396, "DofType"=w397) -> ("Offset"=w392:dbl)  [unwired: 8 in]
            n188 = Add(x=w393, y=w392) -> (x+y=w394:dbl)
            n189 = call "Slider Set Limit.vi"("DofType"=w397, "LBCB Number"=w396, "Value"=w394, "Index"=w395, "error in (no error)"=w391, "Lower/Upper"=Lower_Upper_Select."Upper") -> ("error out"=w390:errorcluster)  [unwired: 9 in]
          }
          frame #2 {
            n190 = call "Slider Set Limit.vi"("DofType"=w404, "LBCB Number"=w403, "Value"=w398, "Index"=w402, "error in (no error)"=w401, "Lower/Upper"=Lower_Upper_Select."Lower") -> ("error out"=w400:errorcluster)  [unwired: 9 in]
          }
          frame #3 {
            n191 = call "Slider Set Limit.vi"("DofType"=w411, "LBCB Number"=w410, "Value"=w405, "Index"=w409, "error in (no error)"=w408, "Lower/Upper"=Lower_Upper_Select."Upper") -> ("error out"=w407:errorcluster)  [unwired: 9 in]
          }
        }
        n192 = Enqueue Element(queue=w366, element=T4 {"Change State"=enum."Limits", "LBCB Number"=enum."LBCB1"}, error in (no error)=w365) -> (queue out=w364:refnum<queue>, error out=w363:errorcluster)  [unwired: 2 out]
        n193 = Enqueue Element(queue=w370, element=Slider_Messages."Update Display", error in (no error)=w363) -> (queue out=w369:refnum<queue>, error out=w368:errorcluster)  [unwired: 1 in, 1 out]
      }
      event #11 {
        n194 = event-data() -> ("OldVal"=w418:cluster{dbl, dbl, dbl, dbl}, "NewVal"=w417:cluster{dbl, dbl, dbl, dbl})  [unwired: 1 in, 3 out]
        n195 = call "Limit Crossover Check.vi"("NewVal"=w417, "OldVal"=w418) -> ("Value"=w425:dbl, "Index"=w426:i32)
        n196 = local read "LBCB Number"() -> (w427:T2)
        n197 = local read "DofType"() -> (w428:T1)
        n198 = case shown="0, Default" w426 {
          tunnel: w428 -> [w437 w446 w453 w460]
          tunnel: w427 -> [w436 w445 w452 w459]
          tunnel: w425 -> [w433 w442 w447 w454]
          tunnel: 3 ("Index") -> [w435 w444 w451 w458]
          tunnel: w423 -> [w431 w440 w450 w457]
          tunnel: [w430 w439 w449 w456] -> w413
          frame #0 {
            n199 = call "Slider Get Offset.vi"("Index"=w435, "LBCB Number"=w436, "DofType"=w437) -> ("Offset"=w432:dbl)  [unwired: 8 in]
            n200 = Add(x=w433, y=w432) -> (x+y=w434:dbl)
            n201 = call "Slider Set Limit.vi"("DofType"=w437, "LBCB Number"=w436, "Value"=w434, "Index"=w435, "error in (no error)"=w431, "Lower/Upper"=Lower_Upper_Select."Lower") -> ("error out"=w430:errorcluster)  [unwired: 9 in]
          }
          frame #1 {
            n202 = call "Slider Get Offset.vi"("Index"=w444, "LBCB Number"=w445, "DofType"=w446) -> ("Offset"=w441:dbl)  [unwired: 8 in]
            n203 = Add(x=w442, y=w441) -> (x+y=w443:dbl)
            n204 = call "Slider Set Limit.vi"("DofType"=w446, "LBCB Number"=w445, "Value"=w443, "Index"=w444, "error in (no error)"=w440, "Lower/Upper"=Lower_Upper_Select."Upper") -> ("error out"=w439:errorcluster)  [unwired: 9 in]
          }
          frame #2 {
            n205 = call "Slider Set Limit.vi"("DofType"=w453, "LBCB Number"=w452, "Value"=w447, "Index"=w451, "error in (no error)"=w450, "Lower/Upper"=Lower_Upper_Select."Lower") -> ("error out"=w449:errorcluster)  [unwired: 9 in]
          }
          frame #3 {
            n206 = call "Slider Set Limit.vi"("DofType"=w460, "LBCB Number"=w459, "Value"=w454, "Index"=w458, "error in (no error)"=w457, "Lower/Upper"=Lower_Upper_Select."Upper") -> ("error out"=w456:errorcluster)  [unwired: 9 in]
          }
        }
        n207 = Enqueue Element(queue=w415, element=T4 {"Change State"=enum."Limits", "LBCB Number"=enum."LBCB1"}, error in (no error)=w413) -> (queue out=w414:refnum<queue>, error out=w412:errorcluster)  [unwired: 2 out]
        n208 = Enqueue Element(queue=w421, element=Slider_Messages."Update Display", error in (no error)=w412) -> (queue out=w420:refnum<queue>, error out=w419:errorcluster)  [unwired: 1 in, 1 out]
      }
      event #12 {
        n209 = event-data() -> ("OldVal"=w477:cluster{dbl, dbl, dbl, dbl}, "NewVal"=w476:cluster{dbl, dbl, dbl, dbl})  [unwired: 1 in, 3 out]
        n210 = local read "LBCB Number"() -> (w474:T2)
        n211 = call "Limit Crossover Check.vi"("NewVal"=w476, "OldVal"=w477) -> ("Value"=w472:dbl, "Index"=w473:i32)
        n212 = local read "DofType"() -> (w475:T1)
        n213 = case shown="0, Default" w473 {
          tunnel: w475 -> [w486 w495 w502 w509]
          tunnel: w474 -> [w485 w494 w501 w508]
          tunnel: w472 -> [w482 w491 w496 w503]
          tunnel: 4 ("Index") -> [w484 w493 w500 w507]
          tunnel: w470 -> [w480 w489 w499 w506]
          tunnel: [w479 w488 w498 w505] -> w462
          frame #0 {
            n214 = call "Slider Get Offset.vi"("Index"=w484, "LBCB Number"=w485, "DofType"=w486) -> ("Offset"=w481:dbl)  [unwired: 8 in]
            n215 = Add(x=w482, y=w481) -> (x+y=w483:dbl)
            n216 = call "Slider Set Limit.vi"("DofType"=w486, "LBCB Number"=w485, "Value"=w483, "Index"=w484, "error in (no error)"=w480, "Lower/Upper"=Lower_Upper_Select."Lower") -> ("error out"=w479:errorcluster)  [unwired: 9 in]
          }
          frame #1 {
            n217 = call "Slider Get Offset.vi"("Index"=w493, "LBCB Number"=w494, "DofType"=w495) -> ("Offset"=w490:dbl)  [unwired: 8 in]
            n218 = Add(x=w491, y=w490) -> (x+y=w492:dbl)
            n219 = call "Slider Set Limit.vi"("DofType"=w495, "LBCB Number"=w494, "Value"=w492, "Index"=w493, "error in (no error)"=w489, "Lower/Upper"=Lower_Upper_Select."Upper") -> ("error out"=w488:errorcluster)  [unwired: 9 in]
          }
          frame #2 {
            n220 = call "Slider Set Limit.vi"("DofType"=w502, "LBCB Number"=w501, "Value"=w496, "Index"=w500, "error in (no error)"=w499, "Lower/Upper"=Lower_Upper_Select."Lower") -> ("error out"=w498:errorcluster)  [unwired: 9 in]
          }
          frame #3 {
            n221 = call "Slider Set Limit.vi"("DofType"=w509, "LBCB Number"=w508, "Value"=w503, "Index"=w507, "error in (no error)"=w506, "Lower/Upper"=Lower_Upper_Select."Upper") -> ("error out"=w505:errorcluster)  [unwired: 9 in]
          }
        }
        n222 = Enqueue Element(queue=w464, element=T4 {"Change State"=enum."Limits", "LBCB Number"=enum."LBCB1"}, error in (no error)=w462) -> (queue out=w463:refnum<queue>, error out=w461:errorcluster)  [unwired: 2 out]
        n223 = Enqueue Element(queue=w468, element=Slider_Messages."Update Display", error in (no error)=w461) -> (queue out=w467:refnum<queue>, error out=w466:errorcluster)  [unwired: 1 in, 1 out]
      }
      event #13 {
        n224 = event-data() -> ("OldVal"=w526:cluster{dbl, dbl, dbl, dbl}, "NewVal"=w525:cluster{dbl, dbl, dbl, dbl})  [unwired: 1 in, 3 out]
        n225 = local read "LBCB Number"() -> (w523:T2)
        n226 = call "Limit Crossover Check.vi"("NewVal"=w525, "OldVal"=w526) -> ("Value"=w521:dbl, "Index"=w522:i32)
        n227 = local read "DofType"() -> (w524:T1)
        n228 = case shown="0, Default" w522 {
          tunnel: w524 -> [w535 w544 w551 w558]
          tunnel: w523 -> [w534 w543 w550 w557]
          tunnel: w521 -> [w531 w540 w545 w552]
          tunnel: 5 ("Index") -> [w533 w542 w549 w556]
          tunnel: w519 -> [w529 w538 w548 w555]
          tunnel: [w528 w537 w547 w554] -> w511
          frame #0 {
            n229 = call "Slider Get Offset.vi"("Index"=w533, "LBCB Number"=w534, "DofType"=w535) -> ("Offset"=w530:dbl)  [unwired: 8 in]
            n230 = Add(x=w531, y=w530) -> (x+y=w532:dbl)
            n231 = call "Slider Set Limit.vi"("DofType"=w535, "LBCB Number"=w534, "Value"=w532, "Index"=w533, "error in (no error)"=w529, "Lower/Upper"=Lower_Upper_Select."Lower") -> ("error out"=w528:errorcluster)  [unwired: 9 in]
          }
          frame #1 {
            n232 = call "Slider Get Offset.vi"("Index"=w542, "LBCB Number"=w543, "DofType"=w544) -> ("Offset"=w539:dbl)  [unwired: 8 in]
            n233 = Add(x=w540, y=w539) -> (x+y=w541:dbl)
            n234 = call "Slider Set Limit.vi"("DofType"=w544, "LBCB Number"=w543, "Value"=w541, "Index"=w542, "error in (no error)"=w538, "Lower/Upper"=Lower_Upper_Select."Upper") -> ("error out"=w537:errorcluster)  [unwired: 9 in]
          }
          frame #2 {
            n235 = call "Slider Set Limit.vi"("DofType"=w551, "LBCB Number"=w550, "Value"=w545, "Index"=w549, "error in (no error)"=w548, "Lower/Upper"=Lower_Upper_Select."Lower") -> ("error out"=w547:errorcluster)  [unwired: 9 in]
          }
          frame #3 {
            n236 = call "Slider Set Limit.vi"("DofType"=w558, "LBCB Number"=w557, "Value"=w552, "Index"=w556, "error in (no error)"=w555, "Lower/Upper"=Lower_Upper_Select."Upper") -> ("error out"=w554:errorcluster)  [unwired: 9 in]
          }
        }
        n237 = Enqueue Element(queue=w513, element=T4 {"Change State"=enum."Limits", "LBCB Number"=enum."LBCB1"}, error in (no error)=w511) -> (queue out=w512:refnum<queue>, error out=w510:errorcluster)  [unwired: 2 out]
        n238 = Enqueue Element(queue=w517, element=Slider_Messages."Update Display", error in (no error)=w510) -> (queue out=w516:refnum<queue>, error out=w515:errorcluster)  [unwired: 1 in, 1 out]
      }
    }
  }
  n239 = while {
    tunnel: w12 -> [w570]
    shift-right: [w567] -> _
    shift-left: w48 -> [w569]
    tunnel: [w562] -> w51
    shift-right: [w559] -> _
    shift-left: w5 -> [w561]
    stop <- w562 stop-if-true
    n240 = Dequeue Element(queue=w569, timeout in ms (-1)=2000, error in (no error)=w561) -> (queue out=w567:refnum<queue>, element=w565:T6, timed out?=w566:bool, error out=w560:errorcluster)
    n241 = Select(t=Slider_Messages."Nothing", s=w566, f=w565) -> (s? t:f=w563:T6)
    n242 = case shown="\"Update Display\"" w563 {
      tunnel: w570 -> [w601 _ _]
      tunnel: [_ TRUE _] -> w562
      tunnel: w560 -> [w572 w633 w635]
      tunnel: [w571 w633 w635] -> w559
      frame #0 {
        n243 = local read "DofType"() -> (w575:T1)
        n244 = local read "LBCB Number"() -> (w574:T2)
        n245 = local read "Limit Slider 1"() -> (w587:T3)
        n246 = local read "Limit Slider 2"() -> (w586:T3)
        n247 = local read "Limit Slider 3"() -> (w585:T3)
        n248 = local read "Limit Slider 4"() -> (w584:T3)
        n249 = local read "Limit Slider 5"() -> (w583:T3)
        n250 = local read "Limit Slider 6"() -> (w582:T3)
        n251 = call "FaultsList.vi"("Limits List Actions"=Faults_List_Actions."Get List") -> ("Fault List"=w576:T12[])  [unwired: 2 in, 8 out]
        n252 = call "Fill Slider Values.vi"("LBCB Number"=w574, "DofType"=w575) -> ("Silder Values"=w573:T15)  [unwired: 9 in]
        n253 = call "Init Slider Boundaries.vi"("DofType"=w575) -> ("Unit Labels"=w579:string[], "Dof Labels"=w580:string[], "Boundaries"=w581:cluster{"[0]":dbl, "[1]":dbl}[])  [unwired: 8 in]
        n254 = call "Fault List 2 Array.vi"("Fault List"=w576, "LBCB Number"=w574, "DofType"=w575) -> ("Faults"=w577:bool[])  [unwired: 8 in]
        n255 = Build Array(w587, w586, w585, w584, w583, w582) -> (w588:T3[])
        n256 = for {
          tunnel: w588 -> [w632] mode=indexing
          tunnel: [w631] -> w602 mode=indexing
          tunnel: w601 -> [w613] mode=indexing
          tunnel: w577 -> [w630] mode=indexing
          tunnel: w581 -> [w629] mode=indexing
          tunnel: w580 -> [w625] mode=indexing
          tunnel: w579 -> [w624] mode=indexing
          tunnel: w573 -> [w623] mode=indexing
          shift-right: [w603] -> w571
          shift-left: w572 -> [w604]
          n257 = Cluster To Array(cluster=w623) -> (array=w622:dbl[])
          n258 = Cluster To Array(cluster=w629) -> (array=w626:dbl[])
          n259 = Index Array(array=w622, index #1=0 ("index"), index #2=1 ("index"), index #3=2 ("index"), index #4=3 ("index"), index #5=4 ("index"), index #6=5 ("index")) -> (element #1=w608:dbl, element #2=w607:dbl, element #3=w610:dbl, element #4=w609:dbl, element #5=w616:dbl, element #6=w614:dbl)
          n260 = Index Array(array=w626, index #1=0 ("index"), index #2=1 ("index")) -> (element #1=w612:dbl, element #2=w611:dbl)
          n261 = Build Array(w610, w609, w608, w607) -> (w606:dbl[])
          n262 = Array To Cluster(array=w606) -> (cluster=w605:T17)
          n263 = Bundle By Name(cluster=w632, "DofLabel"=w625, "Units"=w624, "Fault"=w630, "Global Lo"=w608, "Global Hi"=w607, "Local Lo"=w610, "Local Hi"=w609, "Global Actual"=w616, "Local Actual"=w614, "Slide"=w605) -> (w631:T3)
          n264 = property class="Slide (strict)"(reference=w613, error in=w604, "Scale.Minimum"=w612, "Scale.Maximum"=w611) -> (error out=w603:errorcluster)  [unwired: 1 out]
        }
        n265 = Index Array(array=w602, index #1=0 ("index"), index #2=1 ("index"), index #3=2 ("index"), index #4=3 ("index"), index #5=4 ("index"), index #6=5 ("index")) -> (element #1=w600:T3, element #2=w593:T3, element #3=w592:T3, element #4=w591:T3, element #5=w590:T3, element #6=w589:T3)
        n266 = local write "Limit Slider 1"(w600) -> ()
        n267 = local write "Limit Slider 2"(w593) -> ()
        n268 = local write "Limit Slider 3"(w592) -> ()
        n269 = local write "Limit Slider 4"(w591) -> ()
        n270 = local write "Limit Slider 5"(w590) -> ()
        n271 = local write "Limit Slider 6"(w589) -> ()
      }
      frame #1 {
      }
      frame #2 {
      }
    }
  }
  n272 = Release Queue(queue=w3, error in (no error)=w2) -> (error out=→"error out":errorcluster)  [unwired: 1 in, 2 out]
  n273 = Compound Arithmetic op=AND(w51, w50) -> (w49:bool)
  n274 = flat-sequence {
    tunnel: w49 -> [_]
    tunnel: w10 -> [w638]
    frame #0 {
      n275 = control-ref of="This VI"() -> (w639:refnum<vi>)
      n276 = Release Queue(queue=w638) -> ()  [unwired: 2 in, 3 out]
      n277 = local write "Ok"(FALSE ("Ok")) -> ()
      n278 = invoke class="VI" method="FP.Close"(reference=w639) -> ()  [unwired: 2 in, 3 out]
      n279 = call "NoArgumentsLauncher.vi"("Application"=NoPanelAppTypes."Limits", "Application Launcher Actions"=Launcher_Actions."Stop") -> ()  [unwired: 8 in, 2 out]
    }
  }
